vi "getDeviceName.vi"(8 "error in (no error)":errorcluster, 11 "ScriptEvent in":refnum<class "ScriptEvent.lvclass">) -> (0 "error out":errorcluster, 2 "deviceName":string, 3 "ScriptEvent out":refnum<class "ScriptEvent.lvclass">)   [LabVIEW 2011, in "Tools.lvlib" / "Scripting.lvlib" / "ScriptEvent.lvclass"]
uses:
  ScriptEvent.lvclass
  ScriptEvent.lvclass/ScriptEvent.ctl
  DatabaseHelpers.lvlib
  DatabaseHelpers/DbConnection/DeviceDataBase/deviceDataBase.lvclass
  DatabaseHelpers/Database Objects/Channel/Channel.lvclass
  DatabaseHelpers/Database Objects/DeviceArray/DeviceArray.lvclass
  DatabaseHelpers/Database Objects/device/device.lvclass
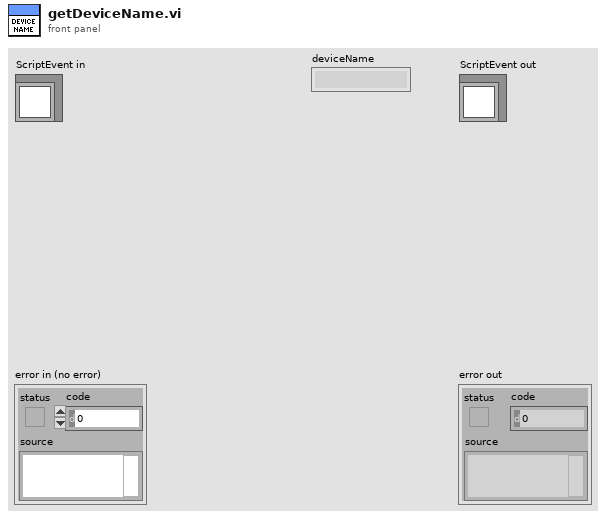
[diagram p1: front panel]
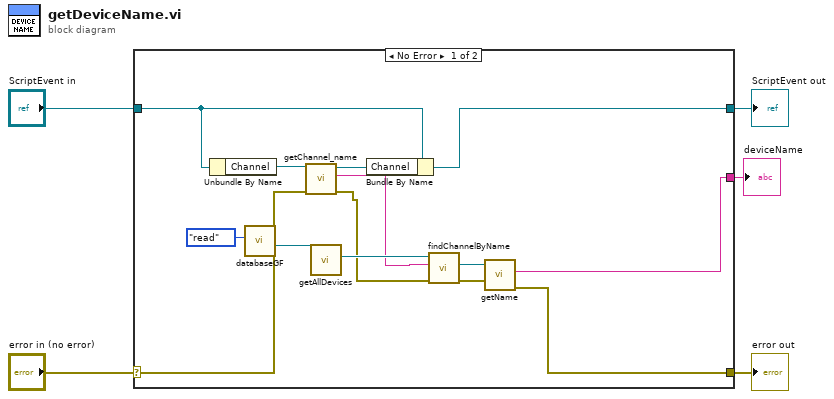
[diagram p0: block diagram]
diagram:
  n1 = case shown="No Error" "error in (no error)" {
    selector: "error in (no error)" -> [w13 w21]
    tunnel: [w6 w21] -> w4
    tunnel: [w18 w20] -> w2
    tunnel: "ScriptEvent in" -> [w19 w20]
    tunnel: [w9 _] -> w1
    frame No Error {
      n2 = Unbundle By Name(w19) -> ("Channel"=w15:refnum<class "Channel.lvclass">)
      n3 = call "databaseGF.vi"("Enum"=enum16{"write", "read"}."read") -> ("deviceDataBase out"=w16:refnum<class "deviceDataBase.lvclass">)  [unwired: 10 in]
      n4 = call "getChannel_name.vi"("error in (no error)"=w13, "Channel.lvclass in"=w15) -> ("error out"=w7:errorcluster, "channel_name"=w11:string, "Channel.lvclass out"=w14:refnum<class "Channel.lvclass">)  [unwired: 7 in]
      n5 = call "getAllDevices.vi"("deviceDataBase in"=w16) -> ("deviceArray.lvclass"=w12:refnum<class "DeviceArray.lvclass">)  [unwired: 8 in, 2 out]
      n6 = Bundle By Name(cluster=w19, "Channel"=w14) -> (w18:refnum<class "ScriptEvent.lvclass">)
      n7 = call "findChannelByName.vi"("error in (no error)"=w7, "channel_name"=w11, "DeviceArray in"=w12) -> ("error out"=w8:errorcluster, "device.lvclass"=w10:refnum<class "device.lvclass">)  [unwired: 4 in, 3 out]
      n8 = call "getName.vi"("error in (no error)"=w8, "device.lvclass in"=w10) -> ("error out"=w6:errorcluster, "name"=w9:string)  [unwired: 7 in, 1 out]
    }
    frame Error {
    }
  }
  "error out" <- w4
  "ScriptEvent out" <- w2
  "deviceName" <- w1
